vi "CreateExecuteCommand.vi"() -> ()   [LabVIEW 2017]
uses:
  <vilib>/Utility/miscctls.llb/LVPointTypeDef.ctl
panel:
  out "Warnings":string
  in  "Path to Template":path=path "C:/Users/Bendethic/Desktop/TestingViscripting/ExecuteCommandTemplate.vi"
  in  "Path to Save":path=path "C:/Users/Bendethic/Desktop/TestingViscripting/ExecuteCommand.vi"
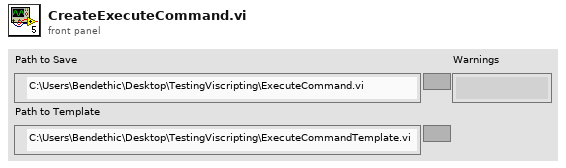
[diagram p1: front panel]
types:
  T1 = typedef "LVPointTypeDef.ctl" = cluster{"Horizontal":i16, "Vertical":i16}
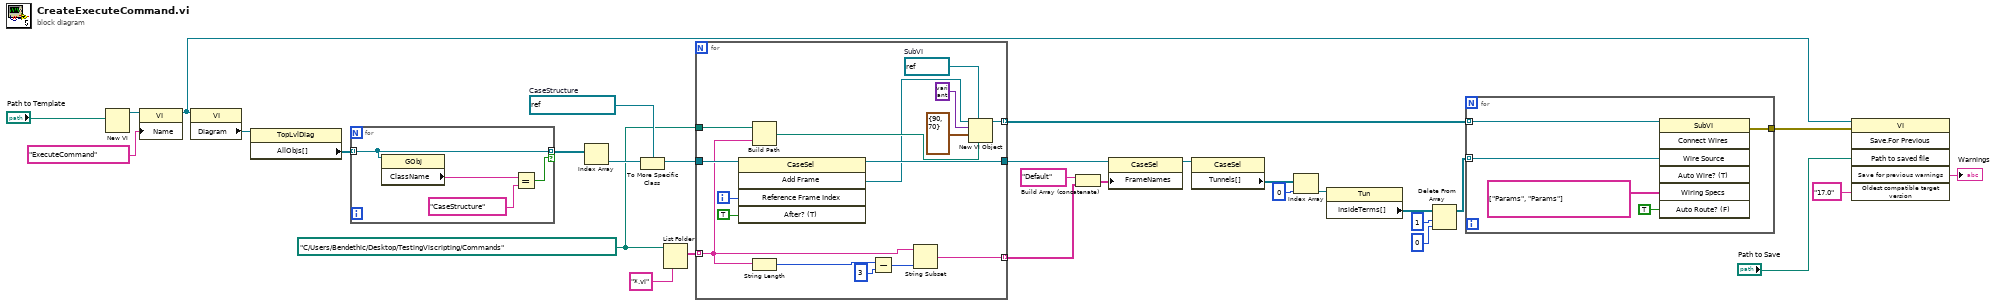
[diagram p0: block diagram]
diagram:
  w18 = path "C:/Users/Bendethic/Desktop/TestingViscripting/Commands" ("path")
  w25 = refnum<vi> refnum  # CaseStructure
  n1 = New VI(10:"Path to Template") -> (3:w29:refnum<vi>)  [unwired: 6 in, 1 out]
  n2 = property class="VI"(reference=w29, "Name"="ExecuteCommand" ("VI Name")) -> (reference out=w5:refnum<vi>)  [unwired: 1 in, 1 out]
  n3 = property class="VI"(reference=w5) -> ("Diagram"=w28:refnum<vi>)  [unwired: 1 in, 2 out]
  n4 = property class="TopLvlDiag"(reference=w28) -> ("AllObjs[]"=w16:refnum<vi>[])  [unwired: 1 in, 2 out]
  n5 = for {
    tunnel: w16 -> [w31] mode=indexing
    tunnel: [w31] -> w27 mode=indexing if=w32
    n6 = property class="GObj"(reference=w31) -> ("ClassName"=w34:string)  [unwired: 1 in, 2 out]
    n7 = Equal?(x=w34, y="CaseStructure") -> (x = y?=w32:bool)
  }
  n8 = Index Array(array=w27) -> (element=w26:refnum<vi>)  [unwired: 1 in]
  n9 = To More Specific Class(target class=w25, reference=w26) -> (specific class reference=w15:refnum<vi>)  [unwired: 1 in, 1 out]
  n10 = List Folder(path=w18, pattern="*.vi") -> (filenames=w23:string[])  [unwired: 2 in, 3 out]
  n11 = for {
    tunnel: w15 -> [w49]
    tunnel: w23 -> [w39] mode=indexing
    tunnel: [w48] -> w17
    tunnel: [w35] -> w22 mode=indexing
    tunnel: w18 -> [w47]
    tunnel: [w40] -> w11 mode=indexing
    i -> [w42]
    w45 = refnum<vi> refnum  # SubVI
    n12 = invoke class="CaseSel" method="Add Frame"(reference=w49, "Reference Frame Index"=w42, "After? (T)"=TRUE) -> (reference out=w48:refnum<vi>, "Add Frame"=w41:refnum<vi>)  [unwired: 2 in, 3 out]
    n13 = Build Path(base path=w47, name or relative path=w39) -> (appended path=w46:path)
    n14 = String Length(string=w39) -> (length=w38:i32)
    n15 = Subtract(x=w38, y=3) -> (x-y=w36:i32)
    n16 = String Subset(string=w39, length (rest)=w36) -> (substring=w35:string)  [unwired: 1 in]
    n17 = New VI Object(vi object class=w45, owner refnum=w41, style=variant, position/next to=T1 {"Horizontal"=90, "Vertical"=70} ("location"), 6:w46) -> (object refnum=w40:refnum<vi>)  [unwired: 3 in, 1 out]
  }
  n18 = Build Array (concatenate)("Default", w22) -> (w21:string[])
  n19 = property class="CaseSel"(reference=w17, "FrameNames"=w21) -> (reference out=w10:refnum<vi>)  [unwired: 1 in, 1 out]
  n20 = property class="CaseSel"(reference=w10) -> ("Tunnels[]"=w12:refnum<vi>[])  [unwired: 1 in, 2 out]
  n21 = Index Array(array=w12, index=0) -> (element=w13:refnum<vi>)
  n22 = property class="Tun"(reference=w13) -> ("InsideTerms[]"=w9:refnum<vi>[])  [unwired: 1 in, 2 out]
  n23 = Delete From Array(array=w9, length=1, index=0) -> (array with subset deleted=w6:refnum<vi>[])  [unwired: 1 out]
  n24 = for {
    tunnel: w11 -> [w55] mode=indexing
    tunnel: w6 -> [w52] mode=indexing
    tunnel: [w51] -> w4
    n25 = invoke class="SubVI" method="Connect Wires"(reference=w55, "Wire Source"=w52, "Wiring Specs"=string[][] [["Params", "Params"]], "Auto Route? (F)"=TRUE) -> (error out=w51:errorcluster)  [unwired: 3 in, 6 out]
  }
  n26 = invoke class="VI" method="Save.For Previous"(reference=w5, error in=w4, "Path to saved file"="Path to Save", "Oldest compatible target version"="17.0" ("Target Version")) -> ("Save for previous warnings"=→"Warnings":string)  [unwired: 2 in, 5 out]
